vi "Read Self Unified Actor DVR.vi"(11 "Actor in":refnum<class "Actor.lvclass">) -> (2 "Self Unified Actor DVR":refnum<data-value>)   [LabVIEW 2020, in "jettl.lvlib" / "Actor.lvclass"]
uses:
  Actor.lvclass
  Unified Actor.ctl
  jettl.lvlib
  Msg/Msg.lvclass
  Msg Set.ctl
  Msg Input/Msg Input.lvclass
  Msg Output/Msg Output.lvclass
  Unified Actor Relation.ctl
  Teller.ctl
  Msg.ctl
  Msgs.ctl
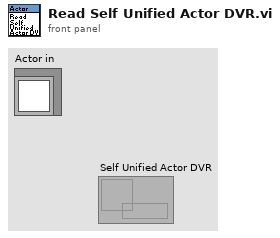
[diagram p1: front panel]
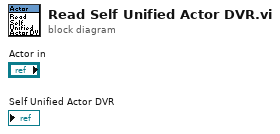
[diagram p0: block diagram]
diagram:
